vi "Coil Calib Select and Get.vi"(4 "error in (no error)":errorcluster, 7 "Magnet ID":string) -> (0 "error out":errorcluster, 2 "File Name":string, 3 "String":string)   [LabVIEW 2020]
doc: "This VI will search for the correct RMPS coil calibration file for the given Magnet ID (Cell name) and return the contents of the file as a string.\nAuthor: Scott Hannahs <sth@magnet.fsu.edu>\nCopyright 2018 Florida State University, All rights reserved."
panel:
  # "Please Select a Calibration File"
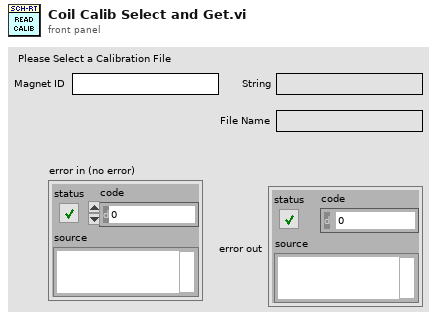
[diagram p1: front panel]
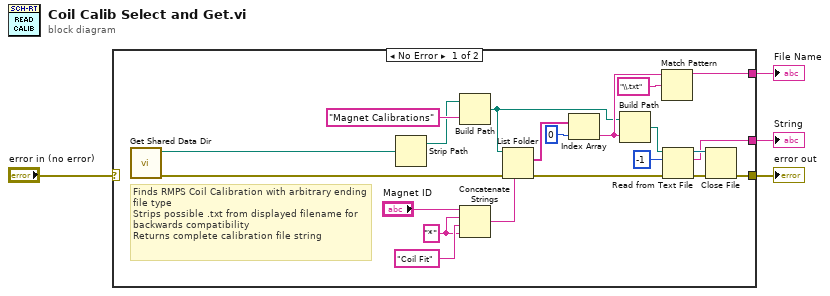
[diagram p0: block diagram]
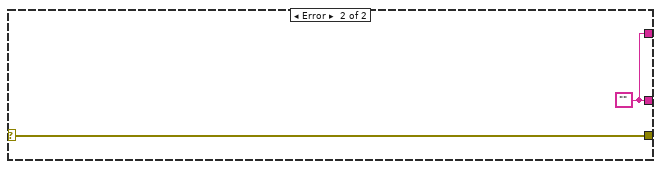
[diagram p2: hidden frame]
diagram:
  n1 = case shown="No Error" "error in (no error)" {
    selector: "error in (no error)" -> [_ w27]
    tunnel: [w10 w27] -> w3
    tunnel: [w9 w26] -> w2
    tunnel: [w8 w26] -> w1
    frame No Error {
      w5 = "*"
      # "Finds RMPS Coil Calibration with arbitrary ending file type\nStrips possible .txt from displayed filename for backwards compatibility\nReturns complete calibration file string"
      n2 = call "Get Shared Data Dir.vi"() -> ("Error Out"=w25:errorcluster, "Data Directory Path"=w16:path)  [unwired: 2 in]
      n3 = Strip Path(path=w16) -> (stripped path=w15:path)  [unwired: 1 out]
      n4 = Build Path(base path=w15, name or relative path="Magnet Calibrations") -> (appended path=w12:path)
      n5 = Concatenate Strings("Magnet ID", w5, "Coil Fit" ("string"), w5) -> (w7:string)
      n6 = List Folder(path=w12, pattern=w7, error in=w25) -> (filenames=w19:string[], error out=w24:errorcluster)  [unwired: 1 in, 2 out]
      n7 = Index Array(array=w19, index=0) -> (element=w21:string)
      n8 = Build Path(base path=w12, name or relative path=w21) -> (appended path=w11:path)
      n9 = Match Pattern(string=w21, regular expression="\\.txt") -> (before substring=w8:string)  [unwired: 1 in, 3 out]
      n10 = Read from Text File(file (use dialog)=w11, count=-1, error in=w24) -> (refnum out=w13:refnum<file>, text=w9:string, error out=w20:errorcluster)  [unwired: 1 in, 1 out]
      n11 = Close File(refnum=w13, error in=w20) -> (error out=w10:errorcluster)  [unwired: 1 out]
    }
    frame Error {
      w26 = ""
    }
  }
  "error out" <- w3
  "String" <- w2
  "File Name" <- w1
